vi "4461 - Create AO waveforms - Multitone.vi"(8 "error in (no error)":errorcluster, 10 "reset signal":bool, 11 "Lockin.DAQ":refnum<class "Lockin.DAQ.lvclass">) -> (0 "error out":errorcluster, 1 "phase out":dbl[](array[numeric]), 2 "AO Array":waveform(dbl)[](array[waveform]), 3 "Lockin.DAQ":refnum<class "Lockin.DAQ.lvclass">)   [LabVIEW 2016, in "Lockin.DAQ.lvclass"]
uses:
  Lockin.DAQ.lvclass
  Typedefs/Sampling.ctl
  Typedefs/Function-enum.ctl
  Lockin.DAQ.lvclass/Lockin.DAQ.ctl
  <vilib>/measure/NI_MABase.lvlib
panel:
  in  "Function":T1[](array[typedef])
  in  "Number of functions":i32
  in  "sampling":T2={"Fs"=204789.0, "#s"=15753}
  in  "Phase (°)":dbl[](array[numeric])
  in  "stop":bool
  in  "f (Hz)":dbl[](array[numeric])
  in  "Amp (V)":dbl[](array[numeric])
  in  "Update graphs?":bool
  out "Waveform Chart":dbl[][](graph)
  out "Waveform Graph":waveform(dbl)[](graph)
  out "Numeric":i32
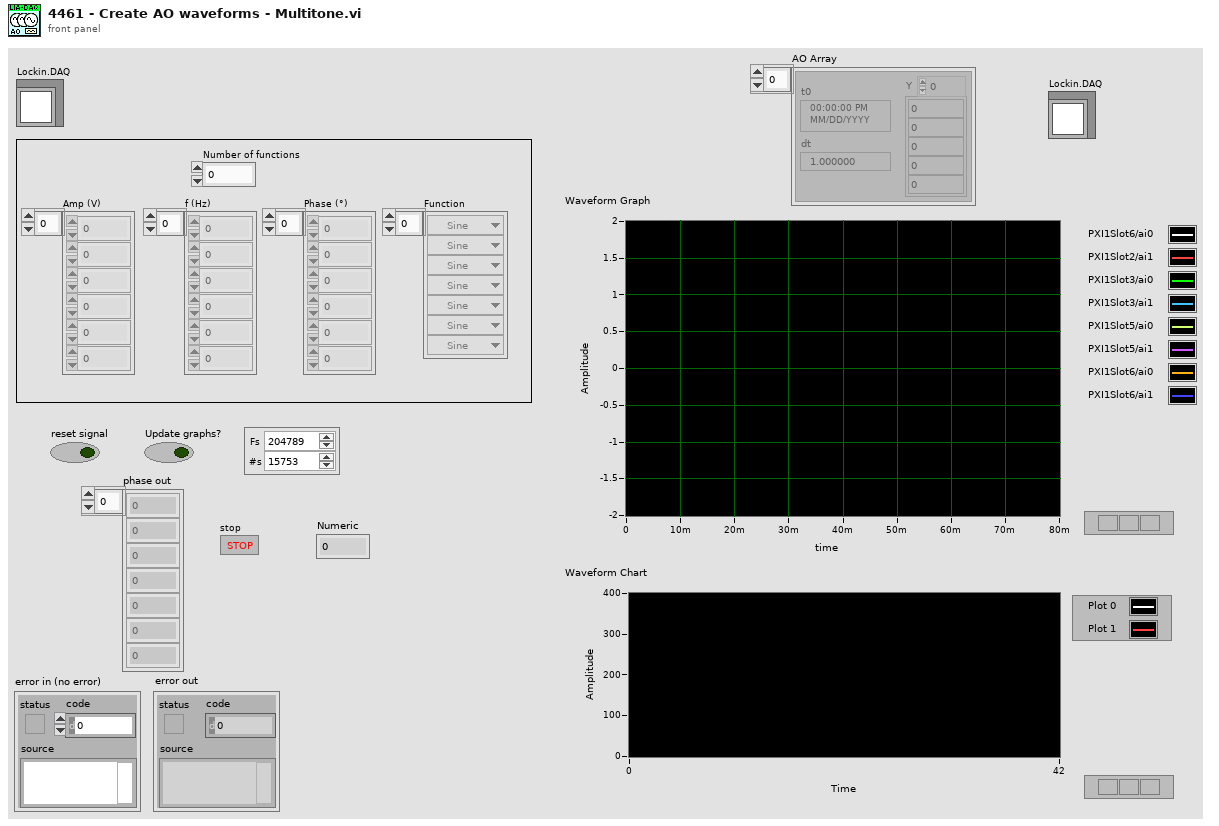
[diagram p1: front panel]
types:
  T1 = typedef "Lockin.DAQ.lvclass/Function-enum.ctl" = enum16{"Sine", "Triangle", "Square", "Sawtooth"}
  T2 = typedef "Lockin.DAQ.lvclass/Sampling.ctl" = cluster{"Fs":dbl, "#s":i32}
  T3 = enum16{"Sine Wave", "Triangle Wave", "Square Wave", "Sawtooth Wave"}
  T4 = typedef "Lockin.DAQ.lvclass/AO-cluster.ctl" = cluster{"Ch":i32[], "Amp (V)":dbl[], "DC (V)":dbl[], "f (Hz)":dbl[], "Phase (°)":dbl[], "Function":T1[], "Sweep?":bool[]}
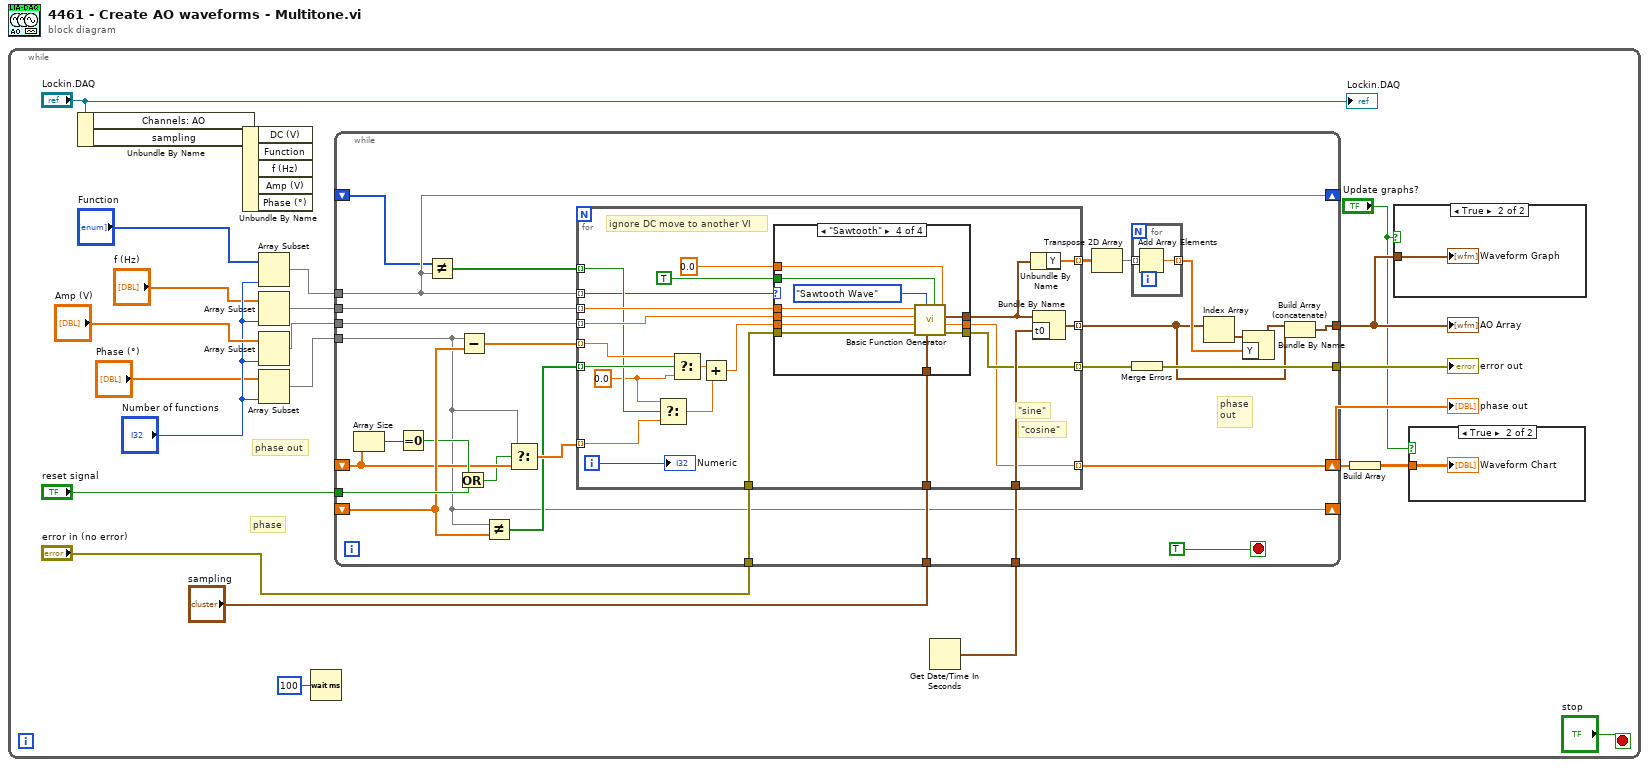
[diagram p0: block diagram]
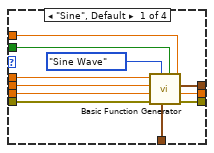
[diagram p4: hidden frame]
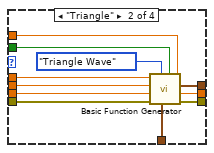
[diagram p5: hidden frame]
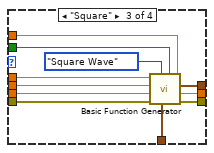
[diagram p6: hidden frame]
diagram:
  n1 = while {
    stop <- "stop" stop-if-true
    # "phase"
    # "phase out"
    n2 = Unbundle By Name("Lockin.DAQ") -> ("Channels: AO"=w13:T4)  [unwired: 1 out]
    n3 = Unbundle By Name(w13) -> ()  [unwired: 5 out]
    n4 = Array Subset(array="Function", length="Number of functions") -> (w5:T1[])  [unwired: 1 in]
    n5 = Array Subset(array="f (Hz)", length="Number of functions") -> (w1:dbl[])  [unwired: 1 in]
    n6 = Array Subset(array="Amp (V)", length="Number of functions") -> (w4:dbl[])  [unwired: 1 in]
    n7 = Array Subset(array="Phase (°)", length="Number of functions") -> (w2:dbl[])  [unwired: 1 in]
    n8 = Wait (ms)(milliseconds to wait=u32 100) -> ()  [unwired: 1 out]
    n9 = Get Date/Time In Seconds() -> (seconds since 1Jan1904=w18:timestamp)
    n10 = while {
      tunnel: w5 -> [w33]
      tunnel: "sampling" -> [w37]
      tunnel: [w28] -> w16
      tunnel: w4 -> [w40]
      tunnel: w2 -> [w36]
      tunnel: w1 -> [w39]
      shift-right: [w36] -> _
      shift-left: _ -> [w46]
      shift-right: [w34] -> w19
      shift-left: _ -> [w42]
      tunnel: w18 -> [w52]
      tunnel: "reset signal" -> [w50]
      tunnel: "error in (no error)" -> [w49]
      tunnel: [w47] -> w17
      shift-right: [w33] -> _
      shift-left: _ -> [w32]
      stop <- TRUE stop-if-true
      # "phase\nout"
      n11 = Array Size(array=w42) -> (size(s)=w51:i32)
      n12 = Equal To 0?(x=w51) -> (x = 0?=w45:bool)
      n13 = Not Equal?(x=w32, y=w33) -> (x != y?=w44:bool[])
      n14 = Or(x=w45, y=w50) -> (x .or. y?=w41:bool)
      n15 = Subtract(x=w36, y=w46) -> (x-y=w35:dbl[])
      n16 = Not Equal?(x=w36, y=w46) -> (x != y?=w38:bool[])
      n17 = Select(t=w36, s=w41, f=w42) -> (s? t:f=w43:dbl[])
      n18 = for {
        tunnel: w33 -> [w60] mode=indexing
        tunnel: w39 -> [w77] mode=indexing
        tunnel: w40 -> [w67] mode=indexing
        tunnel: [w70] -> w25 mode=indexing
        tunnel: w37 -> [w66]
        tunnel: w38 -> [w74] mode=indexing
        tunnel: w35 -> [w75] mode=indexing
        tunnel: w52 -> [w73]
        tunnel: [w68] -> w34 mode=indexing
        tunnel: w49 -> [w58]
        tunnel: [w69] -> w48 mode=indexing
        tunnel: w44 -> [w65] mode=indexing
        tunnel: w43 -> [w63] mode=indexing
        tunnel: [w56] -> w31 mode=indexing
        i -> [w72]
        w64 = 0.0 ("f")
        # "ignore DC move to another VI"
        # "\"cosine\""
        # "\"sine\""
        n19 = Select(t=w64, s=w65, f=w63) -> (s? t:f=w62:dbl)
        n20 = Select(t=w75, s=w74, f=w64) -> (s? t:f=w76:dbl)
        n21 = Add(x=w76, y=w62) -> (x+y=w59:dbl)
        n22 = case shown="\"Sawtooth\"" w60 {
          tunnel: w77 -> [w88 w99 w110 w114]
          tunnel: 0.0 ("AO DC") -> [w87 w98 w109 w118]
          tunnel: [w86 w97 w108 w116] -> w57
          tunnel: TRUE ("reset signal") -> [w78 w89 w100 w119]
          tunnel: w58 -> [w85 w96 w107 w120]
          tunnel: [w84 w95 w106 w121] -> w69
          tunnel: [w83 w94 w105 w115] -> w68
          tunnel: w67 -> [w82 w93 w104 w111]
          tunnel: w59 -> [w81 w92 w103 w112]
          tunnel: w66 -> [w80 w91 w102 w117]
          frame "Sine", Default {
            n23 = call <vilib>:"Basic Function Generator.vi"("offset"=w87, "reset signal"=w78, "sampling info"=w80, "signal type"=T3."Sine Wave", "error in (no error)"=w85, "phase"=w81, "amplitude"=w82, "frequency"=w88) -> ("error out"=w84:errorcluster, "phase out"=w83:dbl, "signal out"=w86:waveform(dbl))  [unwired: 1 in]
          }
          frame "Triangle" {
            n24 = call <vilib>:"Basic Function Generator.vi"("offset"=w98, "reset signal"=w89, "sampling info"=w91, "signal type"=T3."Triangle Wave", "error in (no error)"=w96, "phase"=w92, "amplitude"=w93, "frequency"=w99) -> ("error out"=w95:errorcluster, "phase out"=w94:dbl, "signal out"=w97:waveform(dbl))  [unwired: 1 in]
          }
          frame "Square" {
            n25 = call <vilib>:"Basic Function Generator.vi"("offset"=w109, "reset signal"=w100, "sampling info"=w102, "signal type"=T3."Square Wave", "error in (no error)"=w107, "phase"=w103, "amplitude"=w104, "frequency"=w110) -> ("error out"=w106:errorcluster, "phase out"=w105:dbl, "signal out"=w108:waveform(dbl))  [unwired: 1 in]
          }
          frame "Sawtooth" {
            n26 = call <vilib>:"Basic Function Generator.vi"("offset"=w118, "reset signal"=w119, "sampling info"=w117, "signal type"=T3."Sawtooth Wave", "error in (no error)"=w120, "phase"=w112, "amplitude"=w111, "frequency"=w114) -> ("error out"=w121:errorcluster, "phase out"=w115:dbl, "signal out"=w116:waveform(dbl))  [unwired: 1 in]
          }
        }
        n27 = Unbundle By Name(w57) -> ("Y"=w56:dbl[])
        n28 = Bundle By Name(cluster=w57, "t0"=w73) -> (w70:waveform(dbl))
        "Numeric" <- w72
      }
      n29 = Transpose 2D Array(2D array=w31) -> (transposed array=w30:dbl[][])
      n30 = for {
        tunnel: w30 -> [w55] mode=indexing
        tunnel: [w54] -> w27 mode=indexing
        n31 = Add Array Elements(numeric array=w55) -> (sum=w54:dbl)
      }
      n32 = Merge Errors(w48) -> (w47:errorcluster)
      n33 = Index Array(array=w25) -> (element=w29:waveform(dbl))  [unwired: 1 in]
      n34 = Bundle By Name(cluster=w29, "Y"=w27) -> (w26:waveform(dbl))
      n35 = Build Array (concatenate)(w26, w25) -> (w28:waveform(dbl)[])
    }
    "AO Array" <- w16
    "phase out" <- w19
    "error out" <- w17
    n36 = Build Array(w19) -> (w20:dbl[][])
    n37 = case shown="True" "Update graphs?" {
      tunnel: w16 -> [_ w24]
      frame False {
      }
      frame True {
        "Waveform Graph" <- w24
      }
    }
    n38 = case shown="True" "Update graphs?" {
      tunnel: w20 -> [_ w23]
      frame False {
      }
      frame True {
        "Waveform Chart" <- w23
      }
    }
    "Lockin.DAQ" <- "Lockin.DAQ"
  }
